vi "SUB reverse.vi"(1 "Waveform":waveform(dbl)) -> (0 "Cluster of arrays":cluster{"Y":dbl[], cdb[]})   [LabVIEW 2017]
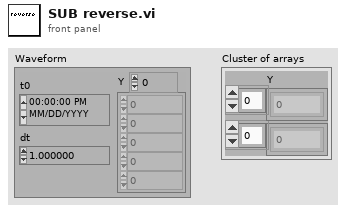
[diagram p1: front panel]
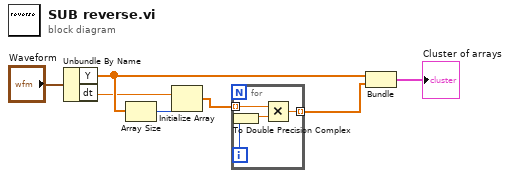
[diagram p0: block diagram]
diagram:
  n1 = Unbundle By Name("Waveform") -> ("Y"=w7:dbl[], "dt"=w5:dbl)
  n2 = Array Size(array=w7) -> (size(s)=w6:i32)
  n3 = Initialize Array(w5, w6) -> (w2:dbl[])
  n4 = for {
    tunnel: w2 -> [w8] mode=indexing
    tunnel: [w11] -> w4 mode=indexing
    i -> [w10]
    n5 = To Double Precision Complex(1:w10) -> (0:w9:cdb)
    n6 = Multiply(x=w8, y=w9) -> (x*y=w11:cdb)
  }
  n7 = Bundle("Y"=w7, w4) -> (→"Cluster of arrays":cluster{"Y":dbl[], cdb[]})  [unwired: 1 in]
